vi "ni579x Read EEPROM Characterization Data.vi"(0 "Register Bus":refnum<class "ni579x Register Bus v1 Host.lvclass">=refnum, 1 "scope":string(combo)="characterization data eeprom", 5 "Device Data Header":T4={"Checksum"=0, "Number of Channels"=0, "Number of Attenuations"=[], "Number of Attenuator Settings"=[], "Number of Gain Settings"=[], "Pointer to Cal Data"=[], "Number of Reserved Bytes"=7, "Number of Frequencies"=[]} {"Checksum" format="%x"}, 11 "Error In":errorcluster) -> (4 "Register Bus (out)":refnum<class "ni579x Register Bus v1 Host.lvclass">, 6 "Characterization Data":T1[](array[typedef]) {"Frequencies [Hz]" format="%#_6p"}, 15 "Error Out":errorcluster)   [LabVIEW 2013]
uses:
  <instrlib>/ni579x/Register Bus/v1/Host/ni579x Register Bus v1 Host.lvclass
  <instrlib>/ni579x/Config/v1/Shared/Types/EEPROM/ni579x EEPROM Device Data Header.ctl
  <instrlib>/ni579x/Config/v1/Shared/Types/ni579x Characterization Data.ctl
  <instrlib>/ni579x/Config/v1/Shared/Types/ni579x IQ Imbalance.ctl
  <instrlib>/ni579x/Config/v1/Shared/Types/ni579x Gain to Attenuation Mapping.ctl
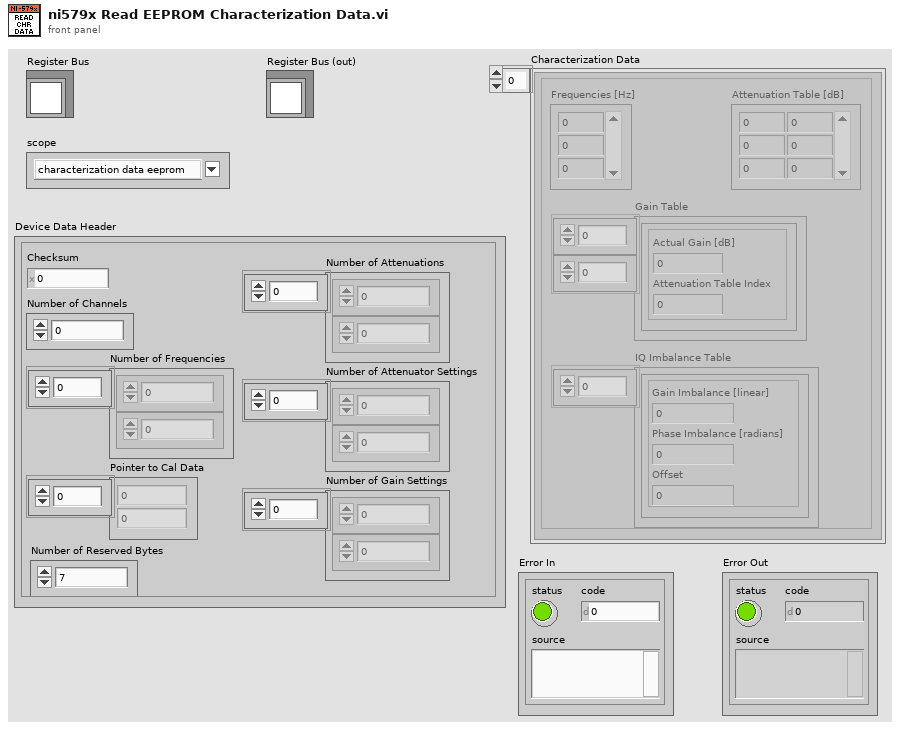
[diagram p1: front panel]
types:
  T1 = typedef "ni579x Characterization Data.ctl" = cluster{"Attenuation Table [dB]":dbl[][], "Frequencies [Hz]":dbl[], "IQ Imbalance Table":T2[], "Gain Table":T3[][]}
  T2 = typedef "ni579x IQ Imbalance.ctl" = cluster{"Gain Imbalance [linear]":dbl, "Phase Imbalance [radians]":dbl, "Offset":cdb}
  T3 = typedef "ni579x Gain to Attenuation Mapping.ctl" = cluster{"Actual Gain [dB]":dbl, "Attenuation Table Index":i32}
  T4 = typedef "ni579x EEPROM Device Data Header.ctl" = cluster{"Checksum":u32, "Number of Channels":u8, "Number of Attenuations":u16[], "Number of Attenuator Settings":u8[], "Number of Gain Settings":u8[], "Pointer to Cal Data":u32[], "Number of Reserved Bytes":i32, "Number of Frequencies":u16[]}
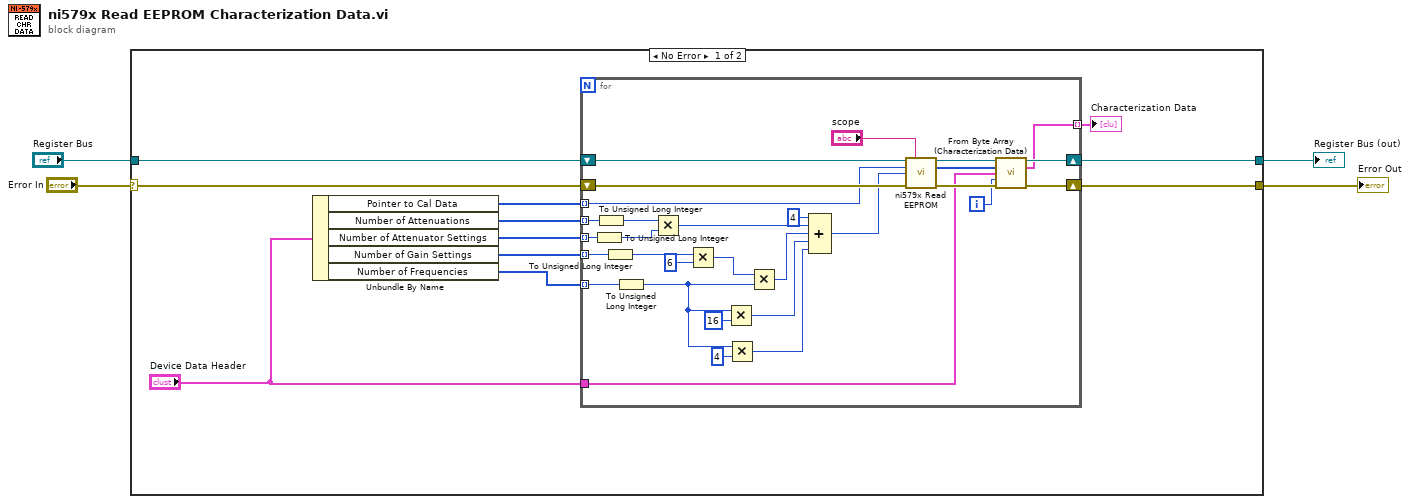
[diagram p0: block diagram]
diagram:
  n1 = case shown="No Error" "Error In" {
    selector: "Error In" -> [w14 w45]
    tunnel: [w12 w45] -> w1
    tunnel: "Register Bus" -> [w15 w46]
    tunnel: [w13 w46] -> w2
    frame No Error {
      n2 = Unbundle By Name("Device Data Header") -> ("Pointer to Cal Data"=w11:u32[], "Number of Attenuations"=w10:u16[], "Number of Attenuator Settings"=w9:u8[], "Number of Gain Settings"=w8:u8[], "Number of Frequencies"=w7:u16[])
      n3 = for {
        tunnel: w11 -> [w41] mode=indexing
        tunnel: w10 -> [w40] mode=indexing
        tunnel: w9 -> [w39] mode=indexing
        tunnel: w8 -> [w38] mode=indexing
        tunnel: w7 -> [w35] mode=indexing
        shift-right: [w28] -> w12
        shift-left: w14 -> [w43]
        shift-right: [w26] -> w13
        shift-left: w15 -> [w44]
        tunnel: "Device Data Header" -> [w25]
        tunnel: [w24] -> w5 mode=indexing
        i -> [w23]
        n4 = To Unsigned Long Integer(number=w39) -> (unsigned 32bit integer=w20:u32)
        n5 = To Unsigned Long Integer(number=w40) -> (unsigned 32bit integer=w21:u32)
        n6 = To Unsigned Long Integer(number=w38) -> (unsigned 32bit integer=w19:u32)
        n7 = To Unsigned Long Integer(number=w35) -> (unsigned 32bit integer=w17:u32)
        n8 = Multiply(x=w21, y=w20) -> (x*y=w33:u32)
        n9 = Multiply(x=w19, y=u32 6) -> (x*y=w36:u32)
        n10 = Multiply(x=w17, y=u32 16) -> (x*y=w31:u32)
        n11 = Multiply(x=w17, y=u32 4) -> (x*y=w16:u32)
        n12 = Multiply(x=w36, y=w17) -> (x*y=w32:u32)
        n13 = Compound Arithmetic op=ADD(u32 4 ("value"), w33, w32, w31, w16) -> (w30:u32)
        n14 = call <instrlib>:"ni579x Read EEPROM.vi"("Register Bus"=w44, "scope"="scope", "start address"=w41, "size"=w30, "Error In"=w43) -> ("Register Bus (out)"=w26:refnum<class "ni579x Register Bus v1 Host.lvclass">, "data"=w27:u8[], "Error Out"=w29:errorcluster)  [unwired: 8 in]
        n15 = call <instrlib>:"From Byte Array (Characterization Data).vi"("byte array in"=w27, "Device Data Header"=w25, "channel"=w23, "Error In"=w29) -> ("Characterization Data"=w24:T1, "Error Out"=w28:errorcluster)  [unwired: 10 in]
      }
      "Characterization Data" <- w5
    }
    frame Error {
    }
  }
  "Register Bus (out)" <- w2
  "Error Out" <- w1
